vi "osciloscope-1-chan.vi"(0 "COM Port":refnum<visa-resource-name>, 5 "Baud Rate (BPS)":u32=9600, 7 "Sampling Frequency (Hz)":sgl, 9 "Refresh Button":bool, 11 "Stop Button":bool, 12 "Time Domain (Block Size)":u16(knob) scale=4.0..10.0, 13 "Frequency Domain (Block Size)":u16(knob) scale=4.0..10.0, 14 "Decimation Factor":u8=1 min=1 max=100) -> (4 "Time Domain":waveform(dbl)(graph), 6 "Frequency Domain":cluster{"f0":dbl, "df":dbl, "magnitude":dbl[]}(graph))   [LabVIEW 2023]
uses:
  <vilib>/Analysis/2dsp.llb/Decimate (single shot, DBL).vi
  <vilib>/Instr/_visa.llb/VISA Configure Serial Port (Instr).vi
  <vilib>/express/express analysis/Spectral/Block/exnSpectralBlock spectral measurements peak poly.vi
  <vilib>/express/express analysis/Spectral/Block/exnSpectralBlock spectral measurements peak WFM.vi
  <vilib>/express/express analysis/Spectral/XNode/ExpressSpectralMeasurementsBlockNode.xnode
  <vilib>/Analysis/NI_AALPro.lvlib
panel:
  out "Frerquency Domain Indicator":u32
  out "Time Domain Indicator":u32
  # "1-CHANNEL OSCILOSCOPE"
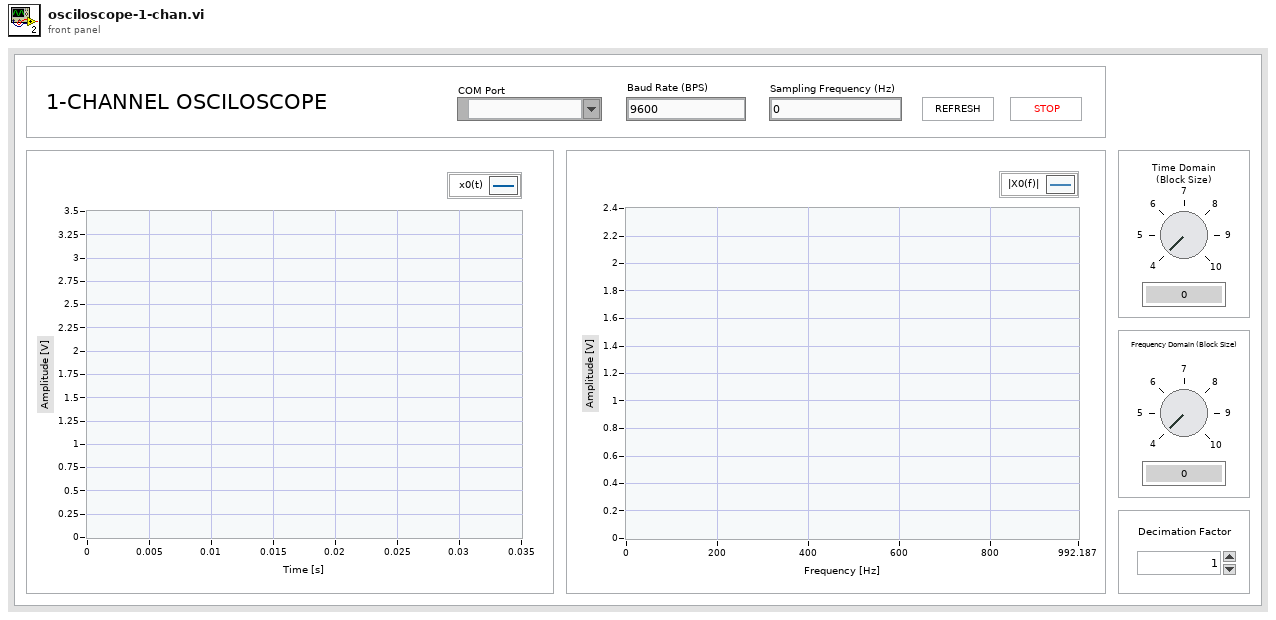
[diagram p1: front panel]
types:
  T1 = cluster{"averaging mode":u16, "weighting mode":u16, "number of averages":u32}
  T2 = cluster{"dB On (F)":bool, "unwrap phase (F)":bool, "convert to degree (F)":bool}
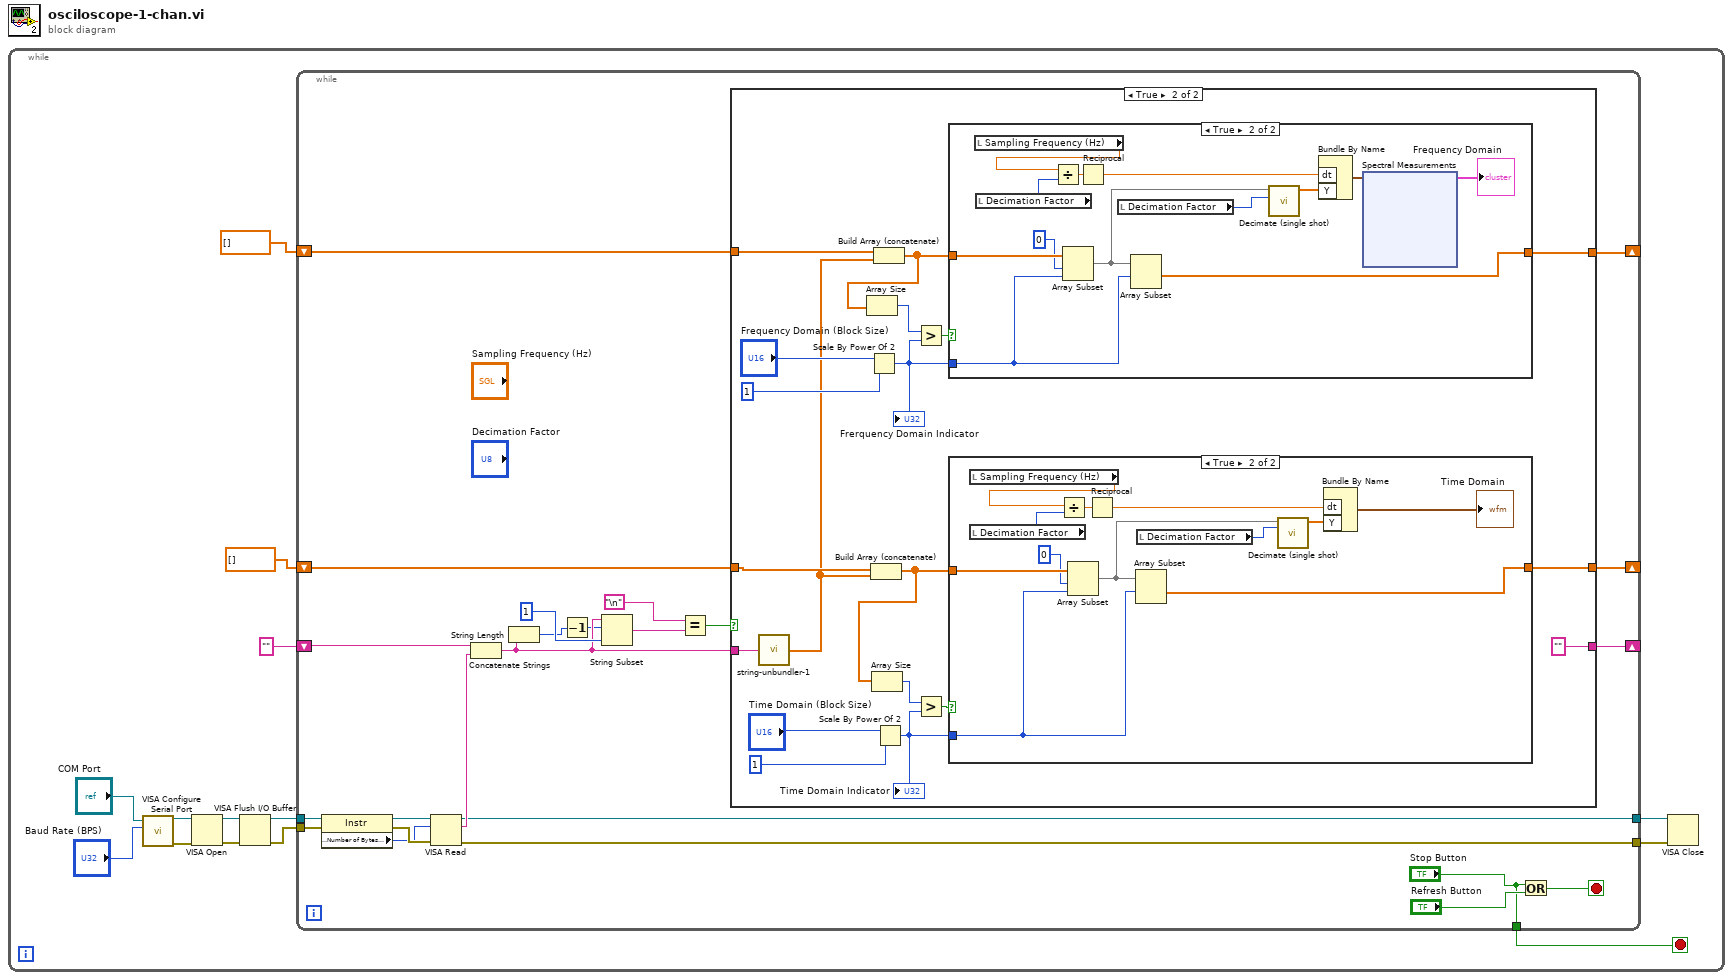
[diagram p0: block diagram]
diagram:
  n1 = while {
    stop <- w1 stop-if-true
    n2 = call-poly "VISA Configure Serial Port"("VISA resource name"="COM Port", "baud rate (9600)"="Baud Rate (BPS)") -> ("VISA resource name out"=w12:refnum<visa-resource-name>, "error out"=w13:errorcluster)  [unwired: 12 in]
    n3 = VISA Open(error in (no error)=w13, VISA resource name=w12) -> (VISA resource name=w11:refnum<visa-resource-name>, error out=w10:errorcluster)  [unwired: 3 in]
    n4 = VISA Flush I/O Buffer(VISA resource name=w11, error in (no error)=w10) -> (VISA resource name out=w14:refnum<visa-resource-name>, error out=w7:errorcluster)  [unwired: 1 in]
    n5 = while {
      tunnel: w14 -> [w38]
      tunnel: w7 -> [w37]
      tunnel: [w20] -> w6
      tunnel: [w21] -> w5
      shift-right: [w31] -> _
      shift-left: "" -> [w32]
      shift-right: [w22] -> _
      shift-left: dbl[] [] -> [w23]
      shift-right: [w18] -> _
      shift-left: dbl[] [] -> [w19]
      tunnel: ["Stop Button"] -> w1
      stop <- w17 stop-if-true
      n6 = property class="Instr"(reference=w38, error in=w37) -> (reference out=w36:refnum<visa-resource-name>, error out=w35:errorcluster, "Serial Settings:Number of Bytes at Serial Port"=w34:u32)
      n7 = VISA Read(VISA resource name=w36, byte count=w34, error in (no error)=w35) -> (VISA resource name out=w21:refnum<visa-resource-name>, read buffer=w33:string, error out=w20:errorcluster)  [unwired: 1 out]
      n8 = Concatenate Strings(w32, w33) -> (w29:string)
      n9 = String Length(string=w29) -> (length=w27:i32)
      n10 = Decrement(x=w27) -> (x-1=w28:i32)
      n11 = String Subset(string=w29, offset (0)=w28, length (rest)=1 ("length (rest)")) -> (substring=w25:string)
      n12 = Equal?(x="\n", y=w25) -> (x = y?=w24:bool)
      n13 = case shown="True" w24 {
        tunnel: w23 -> [w40 w59]
        tunnel: w29 -> [w41 w43]
        tunnel: [w41 ""] -> w31
        tunnel: [w40 w56] -> w22
        tunnel: w19 -> [w39 w55]
        tunnel: [w39 w54] -> w18
        frame False {
        }
        frame True {
          n14 = call "string-unbundler-1.vi"("String"=w43) -> ("Array 1"=w42:dbl[])
          n15 = Scale By Power Of 2(n="Frequency Domain (Block Size)", x=u32 1) -> (x*2^n=w45:u32)
          "Frerquency Domain Indicator" <- w45
          n16 = Build Array (concatenate)(w59, w42) -> (w44:dbl[])
          n17 = Array Size(array=w44) -> (size(s)=w60:i32)
          n18 = Build Array (concatenate)(w55, w42) -> (w46:dbl[])
          n19 = Array Size(array=w46) -> (size(s)=w52:i32)
          n20 = Scale By Power Of 2(n="Time Domain (Block Size)", x=u32 1) -> (x*2^n=w48:u32)
          "Time Domain Indicator" <- w48
          n21 = Greater?(x=w52, y=w45) -> (0:w53:bool)
          n22 = Greater?(x=w60, y=w48) -> (0:w57:bool)
          n23 = case shown="True" w53 {
            tunnel: w46 -> [w61 w74]
            tunnel: [w61 w71] -> w54
            tunnel: w45 -> [_ w62]
            frame False {
            }
            frame True {
              n24 = local read "Sampling Frequency (Hz)"() -> (w65:sgl)
              n25 = local read "Decimation Factor"() -> (w66:u8)
              n26 = Divide(x=w65, y=w66) -> (x/y=w67:sgl)
              n27 = Array Subset(array=w74, index=0, length=w62) -> (w68:dbl[])
              n28 = Reciprocal(x=w67) -> (1/x=w72:sgl)
              n29 = local read "Decimation Factor"() -> (w64:u8)
              n30 = Array Subset(array=w68, index=w62) -> (w71:dbl[])  [unwired: 1 in]
              n31 = call-poly <vilib>:"Decimate (single shot).vi"("decimating factor"=w64, "X"=w68) -> ("Decimated Array"=w69:dbl[])  [unwired: 8 in, 1 out]
              n32 = Bundle By Name("dt"=w72, "Y"=w69) -> (w70:waveform(dbl))  [unwired: 1 in]
              n33 = xnode "Spectral Measurements"("Signals"=w70) -> ("FFT - (Peak)"=→"Frequency Domain":cluster{"f0":dbl, "df":dbl, "magnitude":dbl[]})  [unwired: 1 in, 2 out]
            }
          }
          n34 = case shown="True" w57 {
            tunnel: w44 -> [w85 w97]
            tunnel: w48 -> [_ w95]
            tunnel: [w85 w94] -> w56
            frame False {
            }
            frame True {
              n35 = local read "Sampling Frequency (Hz)"() -> (w89:sgl)
              n36 = local read "Decimation Factor"() -> (w90:u8)
              n37 = Divide(x=w89, y=w90) -> (x/y=w88:sgl)
              n38 = Array Subset(array=w97, index=0, length=w95) -> (w93:dbl[])
              n39 = Reciprocal(x=w88) -> (1/x=w96:sgl)
              n40 = Array Subset(array=w93, index=w95) -> (w94:dbl[])  [unwired: 1 in]
              n41 = local read "Decimation Factor"() -> (w87:u8)
              n42 = call-poly <vilib>:"Decimate (single shot).vi"("decimating factor"=w87, "X"=w93) -> ("Decimated Array"=w92:dbl[])  [unwired: 8 in, 1 out]
              n43 = Bundle By Name("dt"=w96, "Y"=w92) -> (→"Time Domain":waveform(dbl))  [unwired: 1 in]
            }
          }
        }
      }
      n44 = Or(x="Stop Button", y="Refresh Button") -> (x .or. y?=w17:bool)
    }
    n45 = VISA Close(VISA resource name=w5, error in (no error)=w6) -> ()  [unwired: 1 out]
  }
